vi "standardIcon.vi"(8 "Error In":errorcluster, 10 "icon":T1 items=["NoIcon", "Information", "Warning", "Critical", "Question"]) -> (0 "Error Out":errorcluster, 2 "Value":refnum<class "QPixmap.lvclass">)   [LabVIEW 2014, in "QMessageBox.lvclass"]
doc: "LabVIEW-specific documentation is not yet available. See <b>https://doc.qt.io/qt-5/qmessagebox.html#standardIcon</b>"
uses:
  QMessageBox.lvclass
  Qt GUI/QPixmap/QPixmap.lvclass
  Icon.ctl
  LQ Core/LQSerialData/LQSerialData.lvclass/LQSerialData.ctl
  LQ Core/LQ Core.lvlib
  LQ Core/LQSerialData/LQSerialData.lvclass
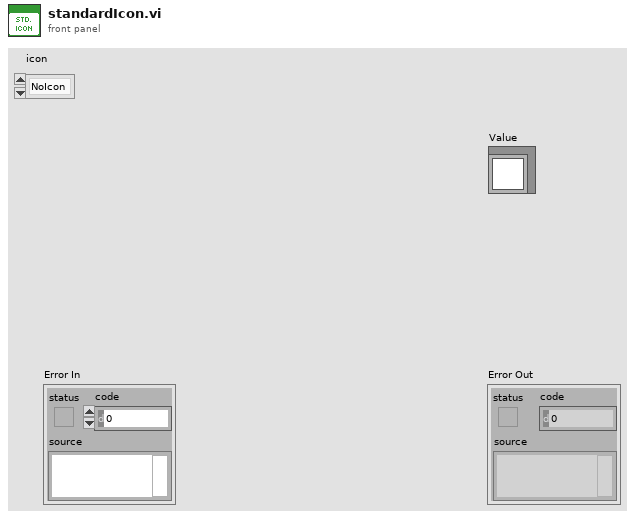
[diagram p1: front panel]
types:
  T1 = typedef "QMessageBox.lvclass/Icon.ctl" = i32
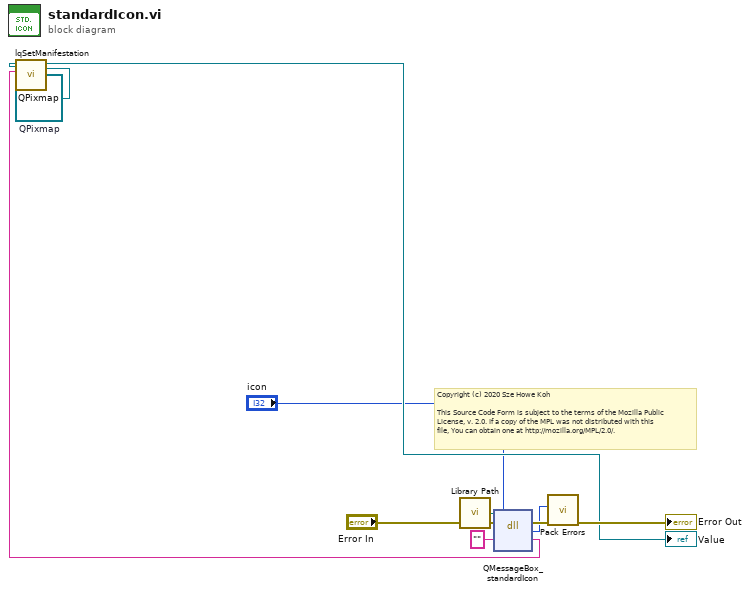
[diagram p0: block diagram]
diagram:
  w2 = refnum<class "QPixmap.lvclass"> refnum  # QPixmap
  # "Copyright (c) 2020 Sze Howe Koh\n\nThis Source Code Form is subject to the terms of the Mozilla Public\nLicense, v. 2.0. If a copy of the MPL was not distributed with this\nfile, You can obtain one at http://mozilla.org/MPL/2.0/."
  n1 = call "Library Path.vi"() -> ("Library Path"=w9:path)
  n2 = dll-call lib="?" fn="QMessageBox_standardIcon"(path in=w9, error in="Error In", "_retVal"="" ("retVal"), "icon"="icon") -> (error out=w7:errorcluster, w5:i32, "_retVal"=w3:string)  [unwired: 2 in, 1 out]
  n3 = call "lqSetManifestation.vi"("Manifestation"=w3, "LQSerialData in"=w2) -> ("LQSerialData out"=→"Value":refnum<class "QPixmap.lvclass">)  [unwired: 8 in, 1 out]
  n4 = call "Pack Errors.vi"("Error In"=w7, "Error Code"=w5) -> ("Error Out"=→"Error Out":errorcluster)  [unwired: 9 in]
